vi "ViewAll.vi"(7 "LabVIEW Web Service Request":refnum<class "Web Request.lvclass">, 10 "ascending":bool=TRUE, 11 "sortMode":u16(ring)=1 items=["Default", "Last Name", "First Name", "Middle Name", "Phone", "Street", "City", "State", "Postal Code", "Favorite"]) -> ()   [LabVIEW 2014]
uses:
  <vilib>/wsapi/Web Request.lvclass
  DataManager/StateStore/Controls/DataFunction.ctl
  <vilib>/wsapi/class/subVIs/Set Integer ESP Variable.vi
  <vilib>/wsapi/class/subVIs/Set Boolean ESP Variable.vi
panel:
  # "Use the Web Service Request input terminal to call the VIs on the Web Services palette. Do not remove it from the connector pane unless you don't need access to the palette."
  # "Each additional control wired to the connector pane will be available as an input in the URL. To include an indicator in terminal-mode output (the default setting), it must also be wired to the connector pane."
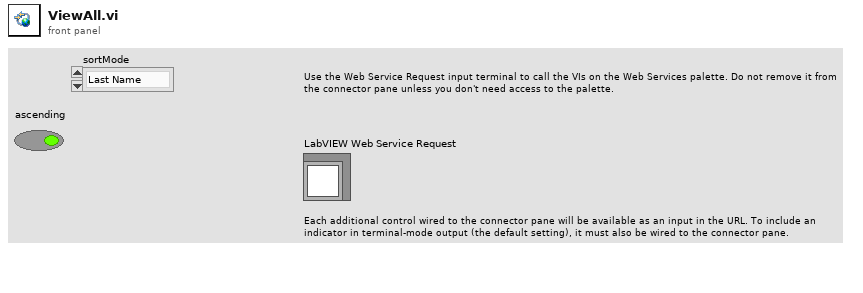
[diagram p1: front panel]
types:
  T1 = typedef "DataFunction.ctl" = enum16{"Initialise", "Release", "Get Data", "Set Data", "Preview Data"}
  T2 = typedef "CData Core Control.ctl" = cluster{"train_data_array":cluster{"uuid":string, "int":i32, "posit_array":cluster{"x":dbl, "y":dbl, "z":dbl}[]}[], "train_control_array":cluster{"uuid":string, "throttle":dbl, "brake":dbl, "horn":dbl, "wait":dbl, "name":string, "mode":string, "dest":string}[], "switch_data_array":cluster{"switch_posit":cluster{"x":dbl, "y":dbl, "z":dbl}, "manual":bool}[], "switch_control_array":cluster{"switch_posit":cluster{"x":dbl, "y":dbl, "z":dbl}, "switch":bool, "invert":bool, "wait":dbl}[]}
  T3 = cluster{"uuid":string, "int":i32, "posit_array":cluster{"x":dbl, "y":dbl, "z":dbl}[]}[]
  T4 = cluster{"uuid":string, "throttle":dbl, "brake":dbl, "horn":dbl, "wait":dbl, "name":string, "mode":string, "dest":string}[]
  T5 = cluster{"uuid":string, "throttle":dbl, "brake":dbl, "horn":dbl, "wait":dbl, "name":string, "mode":string, "dest":string}
  T6 = cluster{"train_data":cluster{"uuid":string, "int":i32, "posit_array":cluster{"x":dbl, "y":dbl, "z":dbl}[]}, "train_control":cluster{"uuid":string, "throttle":dbl, "brake":dbl, "horn":dbl, "wait":dbl, "name":string, "mode":string, "dest":string}}
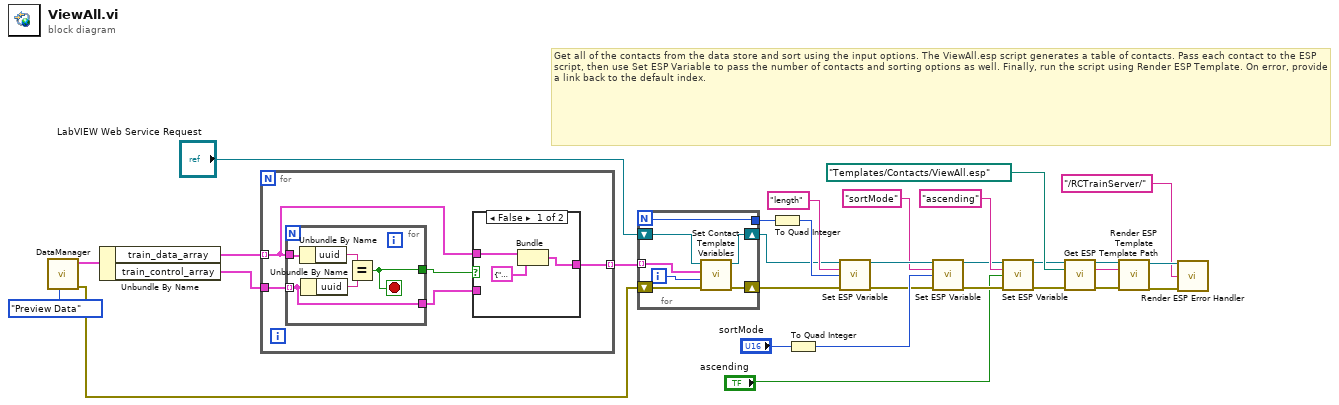
[diagram p0: block diagram]
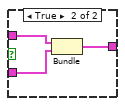
[diagram p2: hidden frame]
diagram:
  # "Get all of the contacts from the data store and sort using the input options. The ViewAll.esp script generates a table of contacts. Pass each contact to the ESP script, then use Set ESP Variable to pass the number of contacts and sorting options as well. Finally, run the script using Render ESP Template. On error, provide a link back to the default index."
  n1 = call "DataManager.vi"("DataFunction"=DataFunction."Preview Data") -> ("error out"=w3:errorcluster, "CData Out"=w2:T2)  [unwired: 9 in]
  n2 = Unbundle By Name(w2) -> ("train_data_array"=w5:T3, "train_control_array"=w4:T4)
  n3 = for {
    tunnel: w5 -> [w33] mode=indexing
    tunnel: w4 -> [w35]
    tunnel: [w31] -> w1 mode=indexing
    n4 = for {
      tunnel: w33 -> [w46]
      tunnel: w35 -> [w42] mode=indexing
      tunnel: [w43] -> w34
      tunnel: [w42] -> w32
      stop <- w43 stop-if-true
      n5 = Unbundle By Name(w46) -> ("uuid"=w44:string)
      n6 = Unbundle By Name(w42) -> ("uuid"=w45:string)
      n7 = Equal?(x=w44, y=w45) -> (x = y?=w43:bool)
    }
    n8 = case shown="False" w34 {
      tunnel: w33 -> [w38 w41]
      tunnel: w32 -> [_ w40]
      tunnel: [w36 w39] -> w31
      frame False {
        n9 = Bundle("train_data"=w38, "train_control"=T5 {"uuid"="", "throttle"=0.0, "brake"=0.0, "horn"=0.0, "wait"=0.0, "name"="", "mode"="", "dest"=""}) -> (w36:T6)  [unwired: 1 in]
      }
      frame True {
        n10 = Bundle("train_data"=w41, "train_control"=w40) -> (w39:T6)  [unwired: 1 in]
      }
    }
  }
  n11 = for {
    N -> [w48]
    tunnel: w1 -> [w47] mode=indexing
    shift-right: [w50] -> w30
    shift-left: w3 -> [w51]
    shift-right: [w49] -> w26
    shift-left: "LabVIEW Web Service Request" -> [w53]
    tunnel: [w48] -> w28
    i -> [w52]
    n12 = call "Set Contact Template Variables.vi"("error in (no error)"=w51, "Index (none)"=w52, "Cluster"=w47, "LabVIEW Web Service Request"=w53) -> ("error out"=w50:errorcluster, "LabVIEW Web Service Request out"=w49:refnum<class "Web Request.lvclass">)  [unwired: 6 in]
  }
  n13 = To Quad Integer(1:w28) -> (0:w27:i64)
  n14 = To Quad Integer(1:"sortMode") -> (0:w14:i64)
  n15 = call-poly <vilib>:"Set ESP Variable.vi"("LabVIEW Web Service Request"=w26, "key"="length", "value"=w27, "error in (no error)"=w30) -> ("LabVIEW Web Service Request out"=w11:refnum<class "Web Request.lvclass">, "error out"=w10:errorcluster)  [unwired: 10 in]
  n16 = call-poly <vilib>:"Set ESP Variable.vi"("LabVIEW Web Service Request"=w11, "key"="sortMode", "value"=w14, "error in (no error)"=w10) -> ("LabVIEW Web Service Request out"=w13:refnum<class "Web Request.lvclass">, "error out"=w17:errorcluster)  [unwired: 10 in]
  n17 = call-poly <vilib>:"Set ESP Variable.vi"("LabVIEW Web Service Request"=w13, "key"="ascending", "value"="ascending", "error in (no error)"=w17) -> ("LabVIEW Web Service Request out"=w8:refnum<class "Web Request.lvclass">, "error out"=w9:errorcluster)  [unwired: 10 in]
  n18 = call "Get ESP Template Path.vi"("LabVIEW Web Service Request"=w8, "Relative Template Path"=path "Templates/Contacts/ViewAll.esp", "error in (no error)"=w9) -> ("LabVIEW Web Service Request out"=w24:refnum<class "Web Request.lvclass">, "Template Name"=w21:string, "error out"=w23:errorcluster)  [unwired: 10 in]
  n19 = call <vilib>:"Render ESP Template.vi"("LabVIEW Web Service Request"=w24, "espName"=w21, "error in (no error)"=w23) -> ("LabVIEW Web Service Request out"=w19:refnum<class "Web Request.lvclass">, "error out"=w20:errorcluster)  [unwired: 11 in]
  n20 = call "Render ESP Error Handler.vi"("LabVIEW Web Service Request"=w19, "Link"="/RCTrainServer/", "error in (no error)"=w20) -> ()  [unwired: 11 in, 2 out]
